vi "enable.vi"(8 "error in (no error)":errorcluster, 11 "Context in":refnum<class "Context.lvclass">) -> (0 "error out":errorcluster, 3 "Context out":refnum<class "Context.lvclass">)   [LabVIEW 2015, in "Context.lvclass"]
uses:
  Context.lvclass
  Model/Model/Model.lvclass
  States/State/State.lvclass
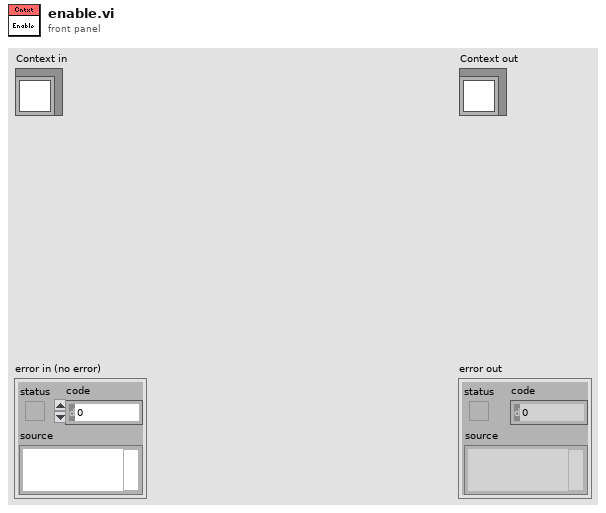
[diagram p1: front panel]
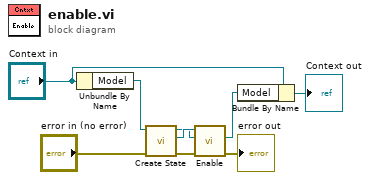
[diagram p0: block diagram]
diagram:
  n1 = Unbundle By Name("Context in") -> ("Model"=w9:refnum<class "Model.lvclass">)
  n2 = call "Create State.vi"("error in (no error)"="error in (no error)", "Model in"=w9) -> ("error out"=w6:errorcluster, "State"=w8:refnum<class "State.lvclass">, "Model out"=w7:refnum<class "Model.lvclass">)  [unwired: 7 in]
  n3 = call-dynamic "Enable.vi"("error in (no error)"=w6, "Model in"=w7, "State in"=w8) -> ("error out"=→"error out":errorcluster, "Model out"=w3:refnum<class "Model.lvclass">)  [unwired: 6 in, 1 out]
  n4 = Bundle By Name(cluster="Context in", "Model"=w3) -> (→"Context out":refnum<class "Context.lvclass">)
